vi "CreateProtectedEvents.vi"(8 "error in (no error)":errorcluster, 11 "DisplayWaveforms":refnum<class "DisplayWaveforms.lvclass">) -> (0 "error out":errorcluster, 3 "DisplayWaveforms out":refnum<class "DisplayWaveforms.lvclass">)   [LabVIEW 2020, in "DisplayWaveform.lvlib" / "DisplayWaveforms.lvclass"]
doc: "---------------------------------------------------------------\nJKI State Machine Objects™\nhttp://jki.net/state-machine-objects/\nCopyright (C) 2005-2015, JKI <info@jki.net>\nALL RIGHTS RESERVEDJKI State Machine Objects (SMO) 1.0.0.5\nJKI - JKI\nCopyright (c) 2016, JKI"
uses:
  DisplayWaveforms.lvclass
  DisplayWaveforms.lvclass/DisplayWaveforms.ctl
  <vilib>/JKI/JKI SMO/SMO.UI/SMO.UI.lvclass
  PumpMeas/TypeDefs/ChartParamsCluster.ctl
  PumpMeas/TypeDefs/NI9208multiplier.ctl
  PumpMeas/TypeDefs/NI9208offset.ctl
  PumpMeas/TypeDefs/NI9205multiplier.ctl
  PumpMeas/TypeDefs/NI9205offset.ctl
panel:
  # "For instructions on how to use the JKI State Machine Objects, examples and video tutorials, visit:\nhttp://jki.net/state-machine-objects/\n\nJKI State Machine Objects™\nhttp://jki.net/state-machine-objects/\nCopyright (C) 2005-2015, JKI <info@jki.net>\nALL RIGHTS RESERVED"
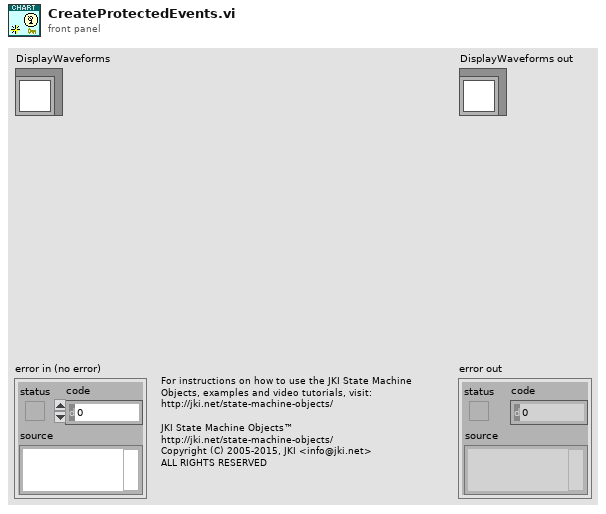
[diagram p1: front panel]
types:
  T1 = typedef "DisplayWaveform.lvlib/DisplayWaveforms.lvclass/PrivateData--Ref.ctl" = refnum<data-value>
  T2 = cluster{"Export Chart":bool, "Export Path Folder":path}
  T3 = typedef "ChartParamsCluster.ctl" = cluster{"Chart ScaleMultipliers":cluster{"WF Xscale Multiplier":dbl, "WF Yscale Multiplier":dbl[]}, "NI9205 Offset":T4, "NI9205 Multipliers":T5, "NI9208 Offset":T6, "NI9208 Multiplier":T7}
  T4 = typedef "NI9205offset.ctl" = cluster{"NI9205 Offset":dbl[]}
  T5 = typedef "NI9205multiplier.ctl" = cluster{"NI9205 Multiplier":dbl[]}
  T6 = typedef "NI9208offset.ctl" = cluster{"NI9208 Offset":dbl[]}
  T7 = typedef "NI9208multiplier.ctl" = cluster{"NI9208 Multiplier":dbl[]}
  T8 = typedef "DisplayWaveform.lvlib/DisplayWaveforms.lvclass/PrivateData--Cluster.ctl" = cluster{"Public Events":T9, "Protected Events":T10, "Data":string, "Dependencies":T11}
  T9 = typedef "DisplayWaveform.lvlib/DisplayWaveforms.lvclass/PublicEvents--Cluster.ctl" = cluster{"Chart Cleared":refnum<user-event>, "Chart Exported":refnum<user-event>, "ChartParams Set":refnum<user-event>}
  T10 = typedef "DisplayWaveform.lvlib/DisplayWaveforms.lvclass/ProtectedEvents--Cluster.ctl" = cluster{"Clear Chart":refnum<user-event>, "Pause Chart":refnum<user-event>, "Update Chart":refnum<user-event>, "Export Chart":refnum<user-event>, "Set ChartParams":refnum<user-event>}
  T11 = typedef "DisplayWaveform.lvlib/DisplayWaveforms.lvclass/Dependencies--Cluster.ctl" = cluster{"New Value":refnum<user-event>}
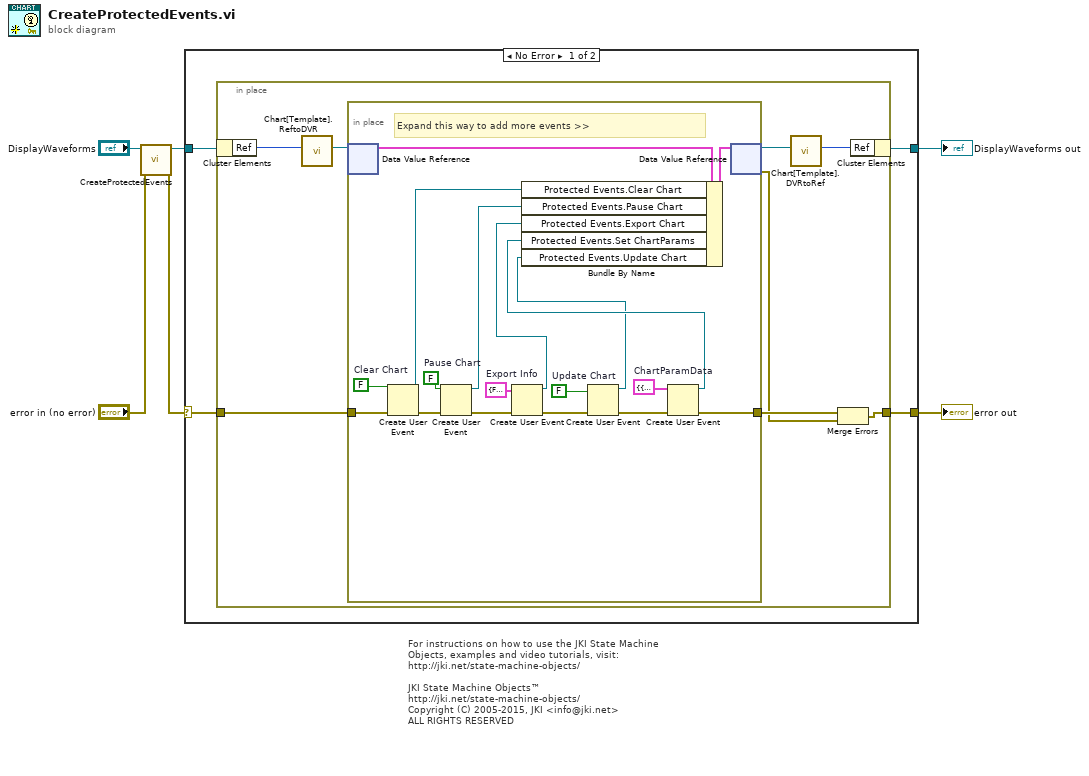
[diagram p0: block diagram]
diagram:
  # "For instructions on how to use the JKI State Machine Objects, examples and video tutorials, visit:\nhttp://jki.net/state-machine-objects/\n\nJKI State Machine Objects™\nhttp://jki.net/state-machine-objects/\nCopyright (C) 2005-2015, JKI <info@jki.net>\nALL RIGHTS RESERVED"
  n1 = call-parent "CreateProtectedEvents.vi"("error in (no error)"="error in (no error)", "SMO"="DisplayWaveforms") -> ("error out"=w1:errorcluster, "SMO out"=w3:refnum<class "DisplayWaveforms.lvclass">)  [unwired: 8 in]
  n2 = case shown="No Error" w1 {
    selector: w1 -> [w8 w38]
    tunnel: [w7 w38] -> w5
    tunnel: [w9 w37] -> w6
    tunnel: w3 -> [w10 w37]
    frame No Error {
      n3 = in-place {
        in-place-border: w8 -> [w18]
        in-place-border: [w15] -> w7
        n4 = in-place-cluster #1(w10) -> ("Ref"=w14:u32)
        n5 = call "Chart[Template].ReftoDVR.vi"("Ref"=w14) -> ("Ref"=w13:T1)  [unwired: 10 in]
        n6 = in-place {
          in-place-border: w18 -> [w35]
          in-place-border: [w28] -> w17
          w20 = T2 {"Export Chart"=FALSE, "Export Path Folder"=path ""}  # Export Info
          w22 = FALSE  # Update Chart
          w25 = cluster{"ChartParams":T3} {"ChartParams"={"Chart ScaleMultipliers"={"WF Xscale Multiplier"=1000.0, "WF Yscale Multiplier"=[]}, "NI9205 Offset"={"NI9205 Offset"=[]}, "NI9205 Multipliers"={"NI9205 Multiplier"=[]}, "NI9208 Offset"={"NI9208 Offset"=[]}, "NI9208 Multiplier"={"NI9208 Multiplier"=[]}}}  # ChartParamData
          w29 = FALSE  # Pause Chart
          w33 = FALSE  # Clear Chart
          # "Expand this way to add more events >>"
          n7 = in-place-dvr #2(w13) -> (w34:T8)  [unwired: 1 out]
          n8 = Create User Event(user event datatype=w33, error in=w35) -> (user event=w32:refnum<user-event>, error out=w31:errorcluster)
          n9 = Create User Event(user event datatype=w29, error in=w31) -> (user event=w30:refnum<user-event>, error out=w26:errorcluster)
          n10 = Create User Event(user event datatype=w20, error in=w26) -> (user event=w19:refnum<user-event>, error out=w24:errorcluster)
          n11 = Create User Event(user event datatype=w22, error in=w24) -> (user event=w21:refnum<user-event>, error out=w23:errorcluster)
          n12 = Create User Event(user event datatype=w25, error in=w23) -> (user event=w27:refnum<user-event>, error out=w28:errorcluster)
          n13 = Bundle By Name(cluster=w34, "Protected Events.Clear Chart"=w32, "Protected Events.Pause Chart"=w30, "Protected Events.Export Chart"=w19, "Protected Events.Set ChartParams"=w27, "Protected Events.Update Chart"=w21) -> (w36:T8)
          n14 = in-place-dvr #2(w36) -> (w12:T1, w16:errorcluster)
        }
        n15 = call "Chart[Template].DVRtoRef.vi"("Ref"=w12) -> ("Ref"=w11:u32)  [unwired: 10 in]
        n16 = Merge Errors(w17, w16) -> (w15:errorcluster)
        n17 = in-place-cluster #1("Ref"=w11) -> (w9:refnum<class "DisplayWaveforms.lvclass">)
      }
    }
    frame Error {
    }
  }
  "error out" <- w5
  "DisplayWaveforms out" <- w6
